vi "control_for.vi"() -> ()   [LabVIEW 2025]
panel:
  out "t":dbl[](array[numeric])
  in  "Boolean":bool
  in  "n_value":i32
  out "Slide":dbl(slide) scale=0.0..100.0
  in  "Array 2 - 1":dbl
  in  "Array 2 - 0":dbl
  out "i_value":i32
  in  "Array 1 -  1":dbl
  in  "Array 1 - 0":dbl
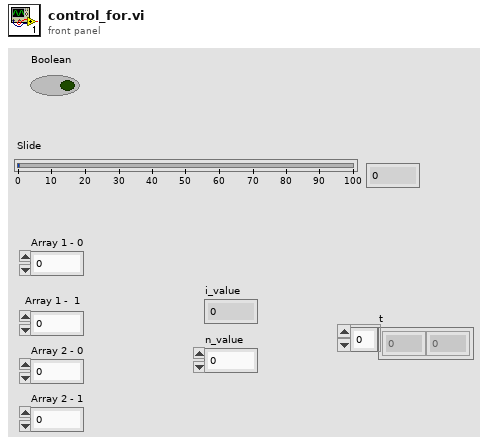
[diagram p1: front panel]
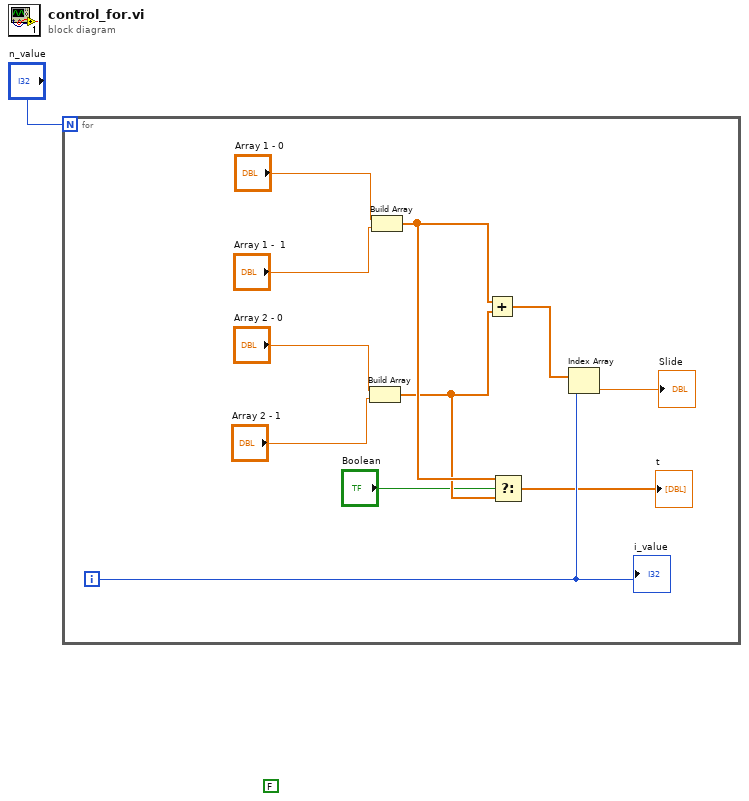
[diagram p0: block diagram]
diagram:
  (unwired) FALSE
  n1 = for {
    N: "n_value" -> [_]
    i -> [w7]
    n2 = Build Array("Array 2 - 0", "Array 2 - 1") -> (w4:dbl[])
    n3 = Build Array("Array 1 - 0", "Array 1 -  1") -> (w5:dbl[])
    n4 = Add(x=w5, y=w4) -> (x+y=w8:dbl[])
    n5 = Select(t=w5, s="Boolean", f=w4) -> (s? t:f=→"t":dbl[])
    n6 = Index Array(array=w8, index=w7) -> (element=→"Slide":dbl)
    "i_value" <- w7
  }
